vi "GlobalVariables.vi"() -> ()   [LabVIEW 2019]
panel:
  out "ESTOP":bool
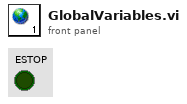
[diagram p1: front panel]
diagram:
